vi "quick approach.vi"(8 "error in":errorcluster, 9 "Destination (steps)":i16, 10 "Numeric":dbl, 11 "Coarse Approach in":refnum<class "Coarse Approach.lvclass">) -> (0 "error out":errorcluster, 1 "Position (steps)":i32, 2 "Amplitude (V rms)":dbl, 3 "Coarse Approach out":refnum<class "Coarse Approach.lvclass">, 4 "x >= y?":bool, 5 "Is moving?":bool)   [LabVIEW 2020, in "Coarse Approach.lvclass"]
uses:
  Coarse Approach.lvclass
  Coarse Approach.lvclass/Coarse Approach.ctl
  Picomotor/Picomotor.lvclass
  Lock-In Amplifier/Lock-In Amplifier.lvclass
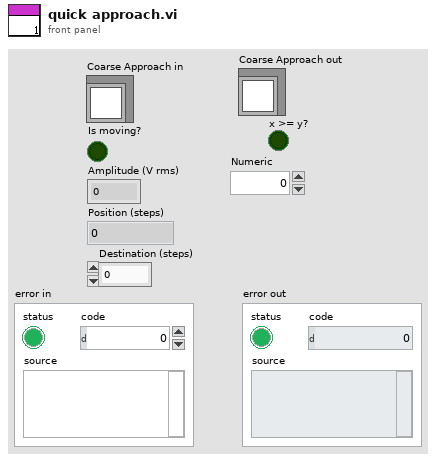
[diagram p1: front panel]
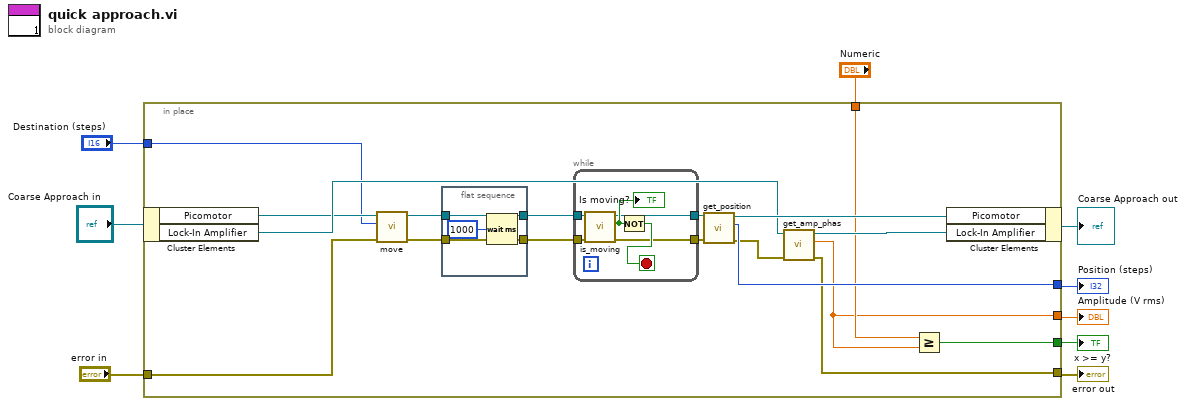
[diagram p0: block diagram]
diagram:
  n1 = in-place {
    in-place-border: "Destination (steps)" -> [w10]
    in-place-border: "error in" -> [w13]
    in-place-border: [w18] -> w5
    in-place-border: [w16] -> w4
    in-place-border: [w23] -> w3
    in-place-border: "Numeric" -> [w17]
    in-place-border: [w15] -> w1
    n2 = in-place-cluster #1("Coarse Approach in") -> ("Picomotor"=w12:refnum<class "Picomotor.lvclass">, "Lock-In Amplifier"=w19:refnum<class "Lock-In Amplifier.lvclass">)
    n3 = call-dynamic "move.vi"("error in"=w13, "Destination (steps)"=w10, "Picomotor in"=w12) -> ("error out"=w14:errorcluster, "Picomotor out"=w11:refnum<class "Picomotor.lvclass">)  [unwired: 7 in]
    n4 = flat-sequence {
      tunnel: w11 -> [w35]
      tunnel: w14 -> [w34]
      tunnel: [w35] -> w27
      tunnel: [w34] -> w26
      frame #0 {
        n5 = Wait (ms)(milliseconds to wait=u32 1000) -> ()  [unwired: 1 out]
      }
    }
    n6 = while {
      tunnel: w27 -> [w31]
      tunnel: w26 -> [w30]
      tunnel: [w29] -> w25
      tunnel: [w28] -> w24
      stop <- w32 stop-if-true
      n7 = call-dynamic "is_moving.vi"("error in (no error)"=w30, "Picomotor in"=w31) -> ("error out"=w28:errorcluster, "Is moving?"=w33:bool, "Picomotor out"=w29:refnum<class "Picomotor.lvclass">)  [unwired: 7 in]
      "Is moving?" <- w33
      n8 = Not(x=w33) -> (.not. x?=w32:bool)
    }
    n9 = call-dynamic "get_position.vi"("error in"=w24, "Picomotor in"=w25) -> ("error out"=w22:errorcluster, "Position"=w23:i32, "Picomotor out"=w21:refnum<class "Picomotor.lvclass">)  [unwired: 7 in]
    n10 = call-dynamic "get_amp_phas.vi"("error in (no error)"=w22, "Lock-In Amplifier in"=w19) -> ("error out"=w18:errorcluster, "Amplitude (V rms)"=w16:dbl, "Lock-In Amplifier out"=w20:refnum<class "Lock-In Amplifier.lvclass">)  [unwired: 6 in, 1 out]
    n11 = Greater Or Equal?(x=w17, y=w16) -> (x >= y?=w15:bool)
    n12 = in-place-cluster #1("Picomotor"=w21, "Lock-In Amplifier"=w20) -> (→"Coarse Approach out":refnum<class "Coarse Approach.lvclass">)
  }
  "error out" <- w5
  "Amplitude (V rms)" <- w4
  "Position (steps)" <- w3
  "x >= y?" <- w1
